vi "SPD.HV_bias Range.vi"(4 "Temperature index":i32, 5 "Continue":refnum<vi>, 6 "deadtime index":i32, 7 "Progress":refnum<vi>, 8 "Error In":errorcluster, 11 "SPD.Stand Ctrl in":T1={"spdDeviceSession"={"spdRef"=0, "connected"=FALSE, "spdName"="", "specification"={"diod case"=enum."default", "type"=enum."Unknown", "frequency"=enum."Unknown"}, "hidSPD.Controller"={"TSet"=0.0, "HV_bias"=0.0, "DDS_stb_code"=0}, "hidSPD.Sturtup Values"={"TSet"=0.0, "HV_bias"=0.0, "DDS_stb_code"=0}}, "DevBSession"={"DevBRef"="", "connected"=FALSE}, "FreqCSession"={"FreqCRef"="", "timeout"=0.0, "Gate"=0.0, "connected"=FALSE}, "8164BSession"={"Connection ID"=refnum, "Connected"=FALSE, "Info"="", "Slots Info"=[]}, "LeCroySession"={"LeCroySession"="", "connected"=FALSE}, "Events"={"DCRTest"=refnum, "Stop"=refnum}, "configFile"={"configFile ref"=refnum, "configFile path"=path "", "equipmentFile ref"=refnum}, "SPD.Meas Grid"={"DateTime"="", "DT"=[], "Insensitivity"=[], "Temprature"=[], "Stb_code"=[], "HV_Bias"=[]}, "SPD.Queues"={"state queue"=refnum}, "Console"=refnum} {"spdDeviceSession"."hidSPD.Sturtup Values"."HV_bias" format="%#_6p, V"; "spdDeviceSession"."hidSPD.Sturtup Values"."TSet" format="%#_6p, DegC"; "spdDeviceSession"."hidSPD.Controller"."HV_bias" format="%#_6p, V"; "spdDeviceSession"."hidSPD.Controller"."TSet" format="%#_6p, DegC"}) -> (0 "Error Out":errorcluster, 1 "done":bool, 2 "Report":string, 3 "SPD.Stand Ctrl out":T1={"spdDeviceSession"={"spdRef"=0, "connected"=FALSE, "spdName"="", "specification"={"diod case"=enum."default", "type"=enum."Unknown", "frequency"=enum."Unknown"}, "hidSPD.Controller"={"TSet"=0.0, "HV_bias"=0.0, "DDS_stb_code"=0}, "hidSPD.Sturtup Values"={"TSet"=0.0, "HV_bias"=0.0, "DDS_stb_code"=0}}, "DevBSession"={"DevBRef"="", "connected"=FALSE}, "FreqCSession"={"FreqCRef"="", "timeout"=0.0, "Gate"=0.0, "connected"=FALSE}, "8164BSession"={"Connection ID"=refnum, "Connected"=FALSE, "Info"="", "Slots Info"=[]}, "LeCroySession"={"LeCroySession"="", "connected"=FALSE}, "Events"={"DCRTest"=refnum, "Stop"=refnum}, "configFile"={"configFile ref"=refnum, "configFile path"=path "", "equipmentFile ref"=refnum}, "SPD.Meas Grid"={"DateTime"="", "DT"=[], "Insensitivity"=[], "Temprature"=[], "Stb_code"=[], "HV_Bias"=[]}, "SPD.Queues"={"state queue"=refnum}, "Console"=refnum} {"spdDeviceSession"."hidSPD.Sturtup Values"."HV_bias" format="%#_6p, V"; "spdDeviceSession"."hidSPD.Sturtup Values"."TSet" format="%#_6p, DegC"; "spdDeviceSession"."hidSPD.Controller"."HV_bias" format="%#_6p, V"; "spdDeviceSession"."hidSPD.Controller"."TSet" format="%#_6p, DegC"})   [LabVIEW 2018]
uses:
  typedefs/SPD.Stand Ctrl.ctl
  Instruments/SPD HID Interface/hidSPDLibForLabView/LibVIs/hidSPD Controls/hidSPD Device Session.ctl
  Instruments/SPD HID Interface/hidSPDLibForLabView/LibVIs/hidSPD Controls/hidSPD.SPD specification.ctl
  Instruments/SPD HID Interface/hidSPDLibForLabView/LibVIs/hidSPD Controls/hidSPD SPD Diod Case.ctl
  Instruments/SPD HID Interface/hidSPDLibForLabView/LibVIs/hidSPD Controls/hidSPD SPD Type.ctl
  Instruments/SPD HID Interface/hidSPDLibForLabView/LibVIs/hidSPD Controls/hidSPD.STB Frequency.ctl
  Instruments/SPD HID Interface/hidSPDLibForLabView/LibVIs/hidSPD Controls/hidSPD Controller.ctl
  Instruments/KC705 DevBoard/typedefs/DevB.Session.ctl
  Instruments/KeySight 53230A/typedefs/FreqC.Session.ctl
  Instruments/KeySight 8164B/KeySight 8164B LAN InstrLib/typedefs/KeySight 8164B control.ctl
  Instruments/LeCroy SDA830/typedefs/LeCroy.Session.ctl
  typedefs/SPD.Events.ctl
  ConfigFile/SPD.Config File ctrl.ctl
  <vilib>/Utility/config.llb/Config Data RefNum.ctl
  typedefs/SPD.Meas Grid.ctl
  typedefs/SPD.Queues.ctl
  typedefs/SPD.Stand state.ctl
  typedefs/SPD.Common HW Setup ctr.ctl
  Instruments/KeySight 8164B/KeySight 8164B LAN InstrLib.lvlib
  <vilib>/Utility/config.llb/NI_LVConfig.lvlib
  Instruments/SPD HID Interface/hidSPDLibForLabView/hidSPDLibForLabView.lvlib
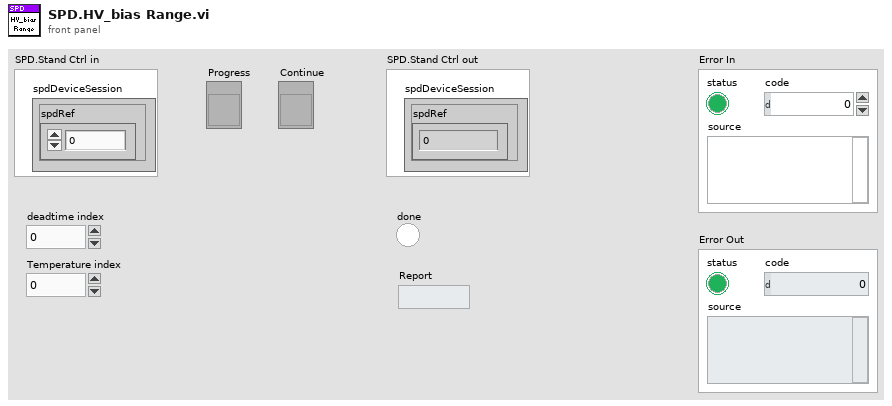
[diagram p1: front panel]
types:
  T1 = typedef "SPD.Stand Ctrl.ctl" = cluster{"spdDeviceSession":T2, "DevBSession":T8, "FreqCSession":T9, "8164BSession":T10, "LeCroySession":T11, "Events":T12, "configFile":T13, "SPD.Meas Grid":T15, "SPD.Queues":T16, "Console":refnum<vi>}
  T2 = typedef "hidSPDLibForLabView.lvlib/hidSPD Device Session.ctl" = cluster{"spdRef":u64, "connected":bool, "spdName":string, "specification":T3, "hidSPD.Controller":T7, "hidSPD.Sturtup Values":T7}
  T3 = typedef "hidSPDLibForLabView.lvlib/hidSPD.SPD specification.ctl" = cluster{"diod case":T4, "type":T5, "frequency":T6}
  T4 = typedef "hidSPDLibForLabView.lvlib/hidSPD SPD Diod Case.ctl" = enum16{"Unknown", "default", "butterfly"}
  T5 = typedef "hidSPDLibForLabView.lvlib/hidSPD SPD Type.ctl" = enum16{"Unknown", "Free Run", "Gate"}
  T6 = typedef "hidSPDLibForLabView.lvlib/hidSPD.STB Frequency.ctl" = enum16{"Unknown", "312", "1250"}
  T7 = typedef "hidSPDLibForLabView.lvlib/hidSPD Controller.ctl" = cluster{"TSet":sgl, "HV_bias":sgl, "DDS_stb_code":u16}
  T8 = typedef "DevB.Session.ctl" = cluster{"DevBRef":refnum<visa-resource-name>, "connected":bool}
  T9 = typedef "FreqC.Session.ctl" = cluster{"FreqCRef":refnum<visa-resource-name>, "timeout":dbl, "Gate":dbl, "connected":bool}
  T10 = typedef "KeySight 8164B LAN InstrLib.lvlib/KeySight 8164B control.ctl" = cluster{"Connection ID":refnum<k5>, "Connected":bool, "Info":string, "Slots Info":string[]}
  T11 = typedef "LeCroy.Session.ctl" = cluster{"LeCroySession":refnum<visa-resource-name>, "connected":bool}
  T12 = typedef "SPD.Events.ctl" = cluster{"DCRTest":refnum<user-event>, "Stop":refnum<user-event>}
  T13 = typedef "SPD.Config File ctrl.ctl" = cluster{"configFile ref":T14, "configFile path":path, "equipmentFile ref":T14}
  T14 = typedef "NI_LVConfig.lvlib/Config Data RefNum.ctl" = refnum<k1>
  T15 = typedef "SPD.Meas Grid.ctl" = cluster{"DateTime":string, "DT":dbl[], "Insensitivity":dbl[], "Temprature":dbl[], "Stb_code":dbl[], "HV_Bias":dbl[][][][]}
  T16 = typedef "SPD.Queues.ctl" = cluster{"state queue":refnum<queue>}
  T17 = typedef "SPD.Common HW Setup ctr.ctl" = cluster{"FS":i32, "TS":i32, "Gate":dbl, "Att1 enable":bool, "Att3 enable":bool, "Att3 Att":dbl, "Scope setup file path":string, "Pset":dbl, "Set Pset":bool}
  T18 = typedef "SPD.HV_Grid Test Params.ctl" = cluster{"FS":i32, "TS":i32, "Initial Step":dbl, "Stop":dbl, "Start":dbl, "Gate":dbl, "Num Of Meas":i32, "max":dbl, "min":dbl, "min delta":dbl, "Num Of intervals":i32}
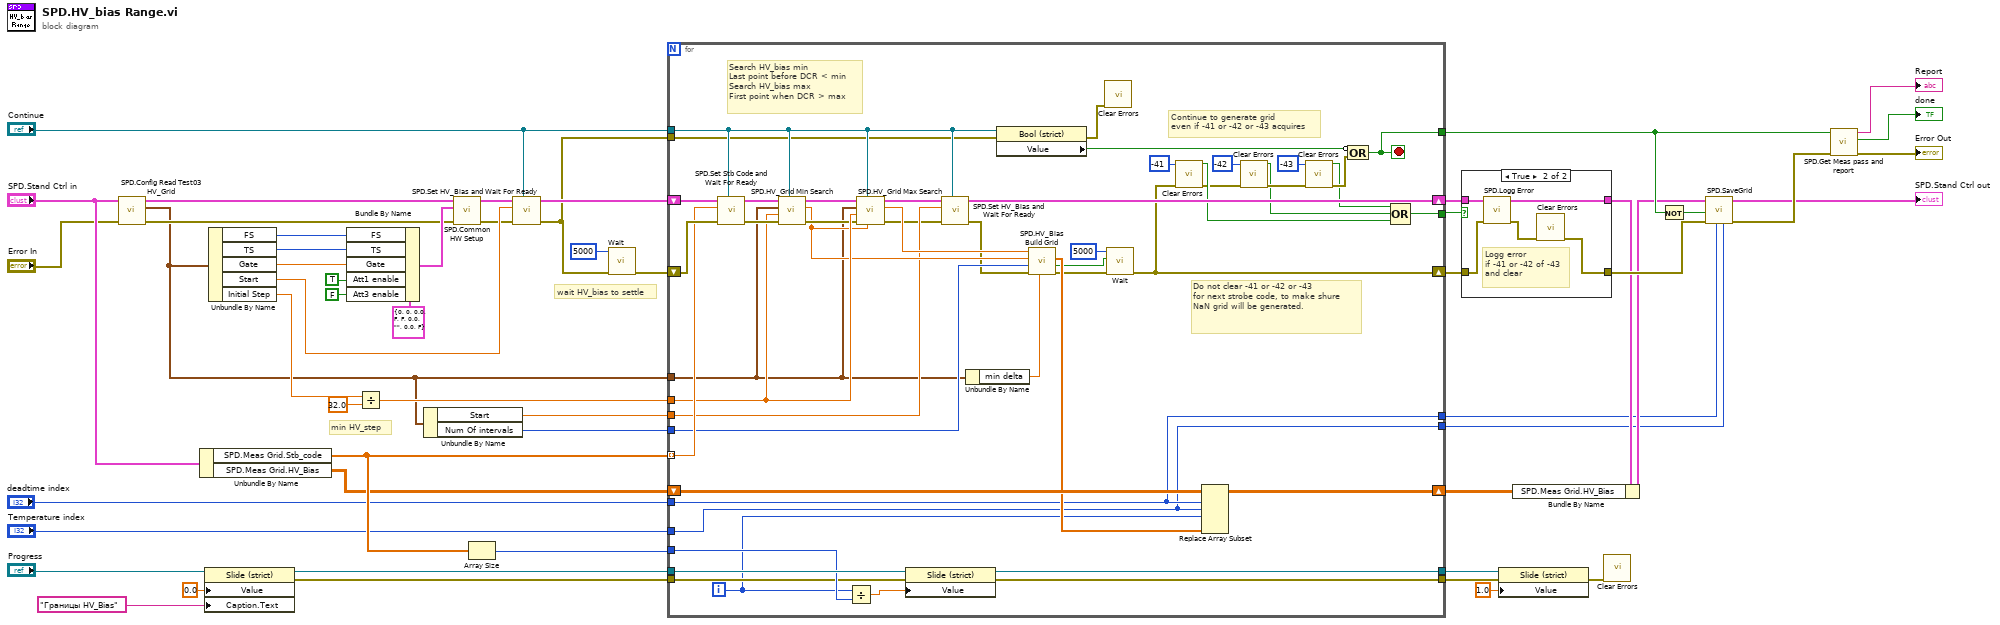
[diagram p0: block diagram]
diagram:
  # "wait HV_bias to settle"
  # "min HV_step"
  n1 = call "SPD.Config Read Test03 HV_Grid.vi"("Error In"="Error In", "SPD.Stand Ctrl in"="SPD.Stand Ctrl in") -> ("Error Out"=w16:errorcluster, "HV_GridParams"=w14:T18, "SPD.Stand Ctrl out"=w17:T1)  [unwired: 7 in]
  n2 = Unbundle By Name("SPD.Stand Ctrl in") -> ("SPD.Meas Grid.Stb_code"=w53:dbl[], "SPD.Meas Grid.HV_Bias"=w52:dbl[][][][])
  n3 = property class="Slide (strict)"(reference="Progress", "Value"=0.0, "Caption.Text"="Границы HV_Bias") -> (reference out=w48:refnum<vi>, error out=w47:errorcluster)  [unwired: 1 in]
  n4 = Unbundle By Name(w14) -> ("FS"=w21:i32, "TS"=w20:i32, "Gate"=w19:dbl, "Start"=w54:dbl, "Initial Step"=w28:dbl)
  n5 = Bundle By Name(cluster=T17 {"FS"=0, "TS"=0, "Gate"=0.0, "Att1 enable"=FALSE, "Att3 enable"=FALSE, "Att3 Att"=0.0, "Scope setup file path"="", "Pset"=0.0, "Set Pset"=FALSE} ("common hw setup"), "FS"=w21, "TS"=w20, "Gate"=w19, "Att1 enable"=TRUE, "Att3 enable"=FALSE) -> (w24:T17)
  n6 = Divide(x=w28, y=32.0) -> (x/y=w37:dbl)
  n7 = Unbundle By Name(w14) -> ("Start"=w36:dbl, "Num Of intervals"=w35:i32)
  n8 = call "SPD.Common HW Setup.vi"("error in (no error)"=w16, "common hw setup"=w24, "SPD.Stand Ctrl in in"=w17) -> ("error out"=w22:errorcluster, "SPD.Stand Ctrl out"=w23:T1)  [unwired: 7 in]
  n9 = Array Size(array=w53) -> (size(s)=w50:i32)
  n10 = call "SPD.Set HV_Bias and Wait For Ready.vi"("Continue"="Continue", "Error In"=w22, "HV_Bias"=w54, "SPD.Stand Ctrl in"=w23) -> ("Error Out"=w29:errorcluster, "SPD.Stand Ctrl out"=w39:T1)  [unwired: 6 in]
  n11 = call "Wait.vi"("error in (no error)"=w29, "milliseconds to wait"=u32 5000) -> ("error out"=w33:errorcluster)  [unwired: 9 in]
  n12 = for {
    tunnel: w53 -> [w102] mode=indexing
    shift-right: [w98] -> w32
    shift-left: w39 -> [w104]
    shift-right: [w60] -> w31
    shift-left: w33 -> [w103]
    tunnel: "Continue" -> [w86]
    tunnel: [w80] -> w8
    tunnel: w50 -> [w99]
    tunnel: w48 -> [w100]
    shift-right: [w96] -> w51
    shift-left: w52 -> [w97]
    tunnel: "Temperature index" -> [w56]
    tunnel: w47 -> [w94]
    tunnel: [w93] -> w45
    tunnel: [w92] -> w44
    tunnel: w14 -> [w65]
    tunnel: w37 -> [w88]
    tunnel: w36 -> [w79]
    tunnel: w35 -> [w78]
    tunnel: [w69] -> w30
    tunnel: w29 -> [w59]
    tunnel: "deadtime index" -> [w57]
    tunnel: [w57] -> w2
    tunnel: [w56] -> w1
    i -> [w58]
    stop <- w80 stop-if-true
    # "Do not clear -41 or -42 or -43 \nfor next strobe code, to make shure \nNaN grid will be generated."
    # "Continue to generate grid\neven if -41 or -42 or -43 acquires"
    # "Search HV_bias min\nLast point before DCR < min\nSearch HV_bias max\nFirst point when DCR > max"
    n13 = call "SPD.Set Stb Code and Wait For Ready.vi"("Continue"=w86, "Error In"=w103, "Strobe code"=w102, "SPD.Stand Ctrl in"=w104) -> ("Error Out"=w90:errorcluster, "SPD.Stand Ctrl out"=w91:T1)  [unwired: 6 in]
    n14 = call "SPD.HV_Grid Min Search.vi"("Continue"=w86, "Error In"=w90, "min step"=w88, "HV_GridParams"=w65, "SPD.Stand Ctrl in"=w91) -> ("Error Out"=w87:errorcluster, "HV_bias min"=w83:dbl, "SPD.Stand Ctrl out"=w89:T1)  [unwired: 3 in, 1 out]
    n15 = Divide(x=w58, y=w99) -> (x/y=w101:dbl)
    n16 = call "SPD.HV_Grid Max Search.vi"("HV_start"=w83, "Continue"=w86, "Error In"=w87, "min step"=w88, "HV_GridParams"=w65, "SPD.Stand Ctrl in"=w89) -> ("Error Out"=w76:errorcluster, "HV_bias max"=w85:dbl, "SPD.Stand Ctrl out"=w84:T1)  [unwired: 2 in, 1 out]
    n17 = property class="Slide (strict)"(reference=w100, error in=w94, "Value"=w101) -> (reference out=w93:refnum<vi>, error out=w92:errorcluster)
    n18 = call "SPD.Set HV_Bias and Wait For Ready.vi"("Continue"=w86, "Error In"=w76, "HV_Bias"=w79, "SPD.Stand Ctrl in"=w84) -> ("Error Out"=w68:errorcluster, "SPD.Stand Ctrl out"=w98:T1)  [unwired: 6 in]
    n19 = Unbundle By Name(w65) -> ("min delta"=w64:dbl)
    n20 = property class="Bool (strict)"(reference=w86, error in=w59) -> (error out=w82:errorcluster, "Value"=w81:bool)  [unwired: 1 out]
    n21 = call "SPD.HV_Bias Build Grid.vi"("min delta V"=w64, "error in (no error)"=w68, "Num Of intervals"=w78, "HV_bias min"=w83, "HV_bias max"=w85) -> ("error out"=w66:errorcluster, "wait before next meas"=w67:bool, "HV_bias Grid"=w95:dbl[])  [unwired: 4 in]
    n22 = call <vilib>:"Clear Errors.vi"("error in (no error)"=w82) -> ()  [unwired: 5 in, 2 out]
    n23 = call "Wait.vi"("error in (no error)"=w66, "wait? (true)"=w67, "milliseconds to wait"=u32 5000) -> ("error out"=w60:errorcluster)  [unwired: 8 in]
    n24 = call <vilib>:"Clear Errors.vi"("error in (no error)"=w60, "specific error code to clear (0: all)"=-41) -> ("error out"=w61:errorcluster, "specific error cleared?"=w62:bool)  [unwired: 4 in]
    n25 = Replace Array Subset(array=w97, new element=w95, index (dim 0)=w57, index (dim 1)=w56, index (dim 2)=w58) -> (w96:dbl[][][][])  [unwired: 1 in]
    n26 = call <vilib>:"Clear Errors.vi"("error in (no error)"=w61, "specific error code to clear (0: all)"=-42) -> ("error out"=w75:errorcluster, "specific error cleared?"=w70:bool)  [unwired: 4 in]
    n27 = call <vilib>:"Clear Errors.vi"("error in (no error)"=w75, "specific error code to clear (0: all)"=-43) -> ("error out"=w74:errorcluster, "specific error cleared?"=w71:bool)  [unwired: 4 in]
    n28 = Compound Arithmetic op=OR(invert w81, w74) -> (w80:bool)
    n29 = Compound Arithmetic op=OR(w71, w70, w62) -> (w69:bool)
  }
  n30 = case shown="True" w30 {
    tunnel: w32 -> [w106 w111]
    tunnel: [w106 w110] -> w6
    tunnel: w31 -> [w105 w109]
    tunnel: [w105 w107] -> w10
    frame False {
    }
    frame True {
      # "Logg error \nif -41 or -42 of -43\nand clear"
      n31 = call "SPD.Logg Error.vi"("Error In"=w109, "SPD.Stand Ctrl in"=w111) -> ("Error Out"=w108:errorcluster, "SPD.Stand Ctrl out"=w110:T1)  [unwired: 8 in]
      n32 = call <vilib>:"Clear Errors.vi"("error in (no error)"=w108) -> ("error out"=w107:errorcluster)  [unwired: 5 in, 1 out]
    }
  }
  n33 = property class="Slide (strict)"(reference=w45, error in=w44, "Value"=1.0) -> (error out=w42:errorcluster)  [unwired: 1 out]
  n34 = Bundle By Name(cluster=w6, "SPD.Meas Grid.HV_Bias"=w51) -> (w5:T1)
  n35 = call <vilib>:"Clear Errors.vi"("error in (no error)"=w42) -> ()  [unwired: 5 in, 2 out]
  n36 = Not(x=w8) -> (.not. x?=w9:bool)
  n37 = call "SPD.SaveGrid.vi"("Temperature index"=w1, "DT index"=w2, "Error In"=w10, "write to file"=w9, "SPD.Stand Ctrl in"=w5) -> ("Error Out"=w7:errorcluster, "SPD.Stand Ctrl out"=→"SPD.Stand Ctrl out":T1)  [unwired: 5 in]
  n38 = call "SPD.Get Meas pass and report.vi"("error in (no error)"=w7, "error or stoped"=w8) -> ("error out"=→"Error Out":errorcluster, "pass"=→"done":bool, "report"=→"Report":string)  [unwired: 7 in]
